vi "Write Interface.vi"(9 "SVW":refnum<class "SharedVariableWrapper.lvclass">, 10 "ConfigInterface":refnum<class "ConfigInterface.lvclass">, 11 "GUI in":refnum<class "GUI.lvclass">) -> (1 "SVW 2":refnum<class "SharedVariableWrapper.lvclass">, 2 "ConfigInterface 2":refnum<class "ConfigInterface.lvclass">, 3 "GUI out":refnum<class "GUI.lvclass">)   [LabVIEW 2019, in "GUI.lvclass"]
uses:
  GUI.lvclass
  ConfigInterface_class/ConfigInterface.lvclass
  SV_Wrap/SharedVariableWrapper.lvclass
  GUI.lvclass/GUI.ctl
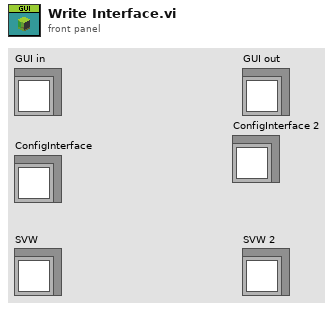
[diagram p1: front panel]
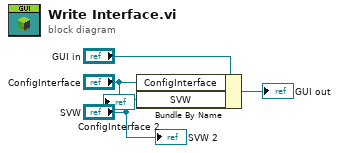
[diagram p0: block diagram]
diagram:
  n1 = Bundle By Name(cluster="GUI in", "ConfigInterface"="ConfigInterface", "SVW"="SVW") -> (→"GUI out":refnum<class "GUI.lvclass">)
  "SVW 2" <- "SVW"
  "ConfigInterface 2" <- "ConfigInterface"
